vi "GetFeedforward_.vi"(11 "scope in":refnum<class "Scope5782_six_channel.lvclass">) -> (1 "values Q":dbl[](array[numeric]), 2 "values I":dbl[](array[numeric]), 3 "scope out":refnum<class "Scope5782_six_channel.lvclass">)   [LabVIEW 2018, in "Scope5782_six_channel.lvclass"]
uses:
  Scope5782_six_channel.lvclass
  Scope5782_six_channel.lvclass/Scope5782_six_channel.ctl
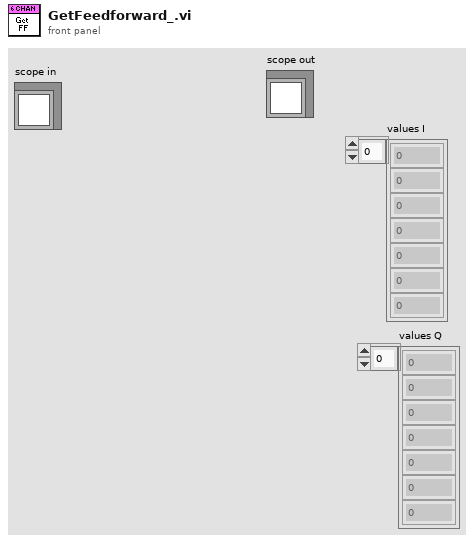
[diagram p1: front panel]
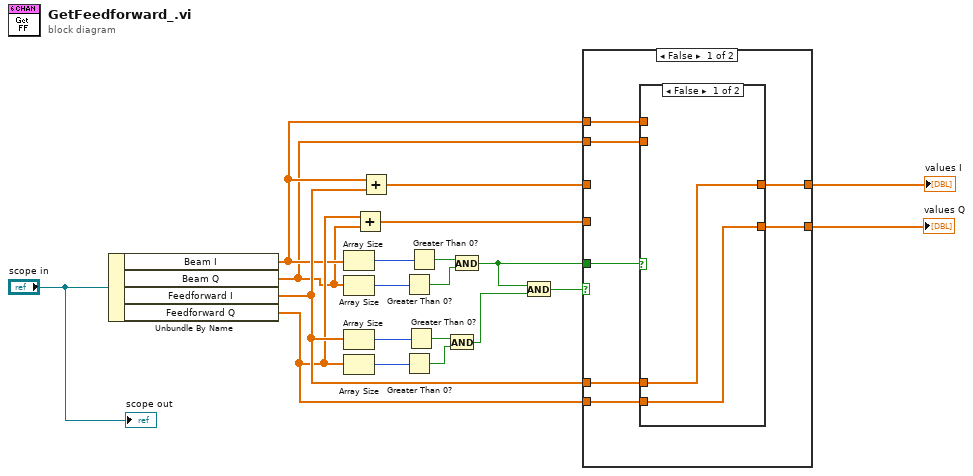
[diagram p0: block diagram]
diagram:
  n1 = Unbundle By Name("scope in") -> ("Beam I"=w3:dbl[], "Beam Q"=w2:dbl[], "Feedforward I"=w5:dbl[], "Feedforward Q"=w4:dbl[])
  n2 = Array Size(array=w3) -> (size(s)=w20:i32)
  n3 = Array Size(array=w2) -> (size(s)=w19:i32)
  n4 = Array Size(array=w5) -> (size(s)=w17:i32)
  n5 = Array Size(array=w4) -> (size(s)=w18:i32)
  n6 = Add(x=w4, y=w2) -> (x+y=w9:dbl[])
  n7 = Add(x=w3, y=w5) -> (x+y=w10:dbl[])
  n8 = Greater Than 0?(x=w19) -> (x > 0?=w15:bool)
  n9 = Greater Than 0?(x=w18) -> (x > 0?=w13:bool)
  n10 = Greater Than 0?(x=w17) -> (x > 0?=w14:bool)
  n11 = Greater Than 0?(x=w20) -> (x > 0?=w16:bool)
  n12 = And(x=w14, y=w13) -> (x .and. y?=w12:bool)
  n13 = And(x=w16, y=w15) -> (x .and. y?=w6:bool)
  n14 = And(x=w6, y=w12) -> (x .and. y?=w11:bool)
  n15 = case shown="False" w11 {
    tunnel: w10 -> [_ w32]
    tunnel: w9 -> [_ w33]
    tunnel: [w21 w33] -> w7
    tunnel: [w22 w32] -> w8
    tunnel: w6 -> [w27 _]
    tunnel: w5 -> [w26 _]
    tunnel: w4 -> [w25 _]
    tunnel: w3 -> [w24 _]
    tunnel: w2 -> [w23 _]
    frame False {
      n16 = case shown="False" w27 {
        tunnel: w26 -> [w29 _]
        tunnel: w25 -> [w28 _]
        tunnel: w24 -> [_ w31]
        tunnel: w23 -> [_ w30]
        tunnel: [w29 w31] -> w22
        tunnel: [w28 w30] -> w21
        frame False {
        }
        frame True {
        }
      }
    }
    frame True {
    }
  }
  "values I" <- w8
  "values Q" <- w7
  "scope out" <- "scope in"
